vi "GetHeadEnumValue.vi"(11 "Head":u8) -> (2 "coerced x":T1, 3 "Head":T1)   [LabVIEW 2022 SP3]
uses:
  Typedefs/PrinterHeads--Enum.ctl
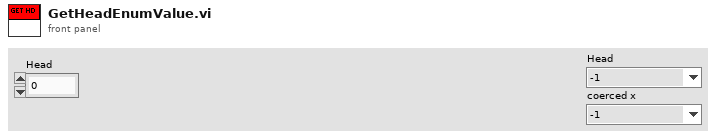
[diagram p1: front panel]
types:
  T1 = typedef "PrinterHeads--Enum.ctl" = enum16{"-1", "1", "2", "3", "4", "5", "6"}
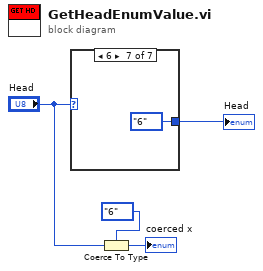
[diagram p0: block diagram]
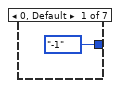
[diagram p2: hidden frame]
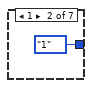
[diagram p3: hidden frame]
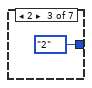
[diagram p4: hidden frame]
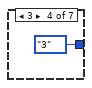
[diagram p5: hidden frame]
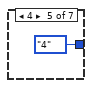
[diagram p6: hidden frame]
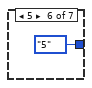
[diagram p7: hidden frame]
diagram:
  n1 = case shown="6" "Head" {
    tunnel: [PrinterHeads--Enum."-1" ("Head") PrinterHeads--Enum."1" ("Head") PrinterHeads--Enum."2" ("Head") PrinterHeads--Enum."3" ("Head") PrinterHeads--Enum."4" ("Head") PrinterHeads--Enum."5" ("Head") PrinterHeads--Enum."6" ("Head")] -> w4
    frame 0, Default {
    }
    frame 1 {
    }
    frame 2 {
    }
    frame 3 {
    }
    frame 4 {
    }
    frame 5 {
    }
    frame 6 {
    }
  }
  "Head" <- w4
  n2 = Coerce To Type(0:"Head", 1:PrinterHeads--Enum."6" ("Head")) -> (2:→"coerced x":T1)
